vi "Display Unicode Strings and Array.vi"() -> ()   [LabVIEW 2009]
panel:
  out "Unicode (hex)":string
  out "2D Array":string[][](array[string])
  out "Unicode":string
  in  "ASCII":string="Hello"
  out "1D Array":string[](array[string])
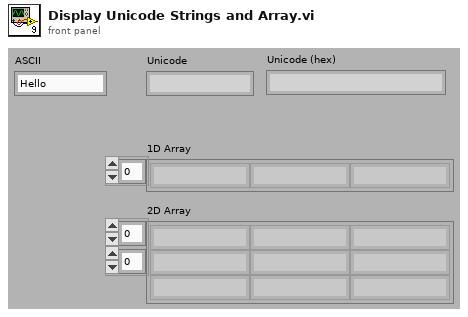
[diagram p1: front panel]
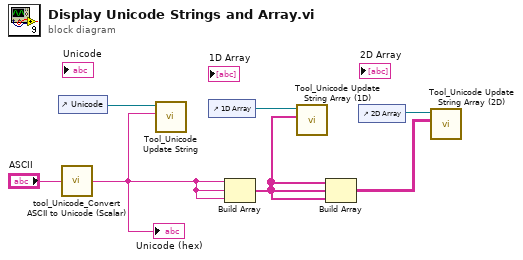
[diagram p0: block diagram]
diagram:
  n1 = control-ref of="Unicode"() -> (w6:refnum<vi>)
  n2 = call "tool_Unicode_Convert ASCII to Unicode (Scalar).vi"("ASCII"="ASCII") -> ("Unicode"=w1:string)  [unwired: 4 in]
  "Unicode (hex)" <- w1
  n3 = call "Tool_Unicode Update String.vi"("String Value"=w1, "String Control Reference"=w6) -> ()  [unwired: 6 in, 2 out]
  n4 = control-ref of="1D Array"() -> (w5:refnum<vi>)
  n5 = Build Array(w1, w1, w1) -> (w4:string[])
  n6 = call "Tool_Unicode Update String Array (1D).vi"("Value"=w4, "String Array (1D) Ref"=w5) -> ()  [unwired: 6 in, 2 out]
  n7 = Build Array(w4, w4, w4) -> (w2:string[][])
  n8 = control-ref of="2D Array"() -> (w3:refnum<vi>)
  n9 = call "Tool_Unicode Update String Array (2D).vi"("Value"=w2, "String Array (2D) Ref"=w3) -> ()  [unwired: 6 in, 2 out]
